vi "create.vi"(8 "error in (no error)":errorcluster, 10 "Port":i32, 11 "IModbusFactory in":refnum<class "IModbusFactory.lvclass">) -> (0 "error out":errorcluster, 2 "IModbus":refnum<class "IModbus.lvclass">, 3 "IModbusFactory out":refnum<class "IModbusFactory.lvclass">)   [LabVIEW 2016, in "IModbusFactory.lvclass"]
uses:
  IModbusFactory.lvclass
  IModbus/IModbus.lvclass
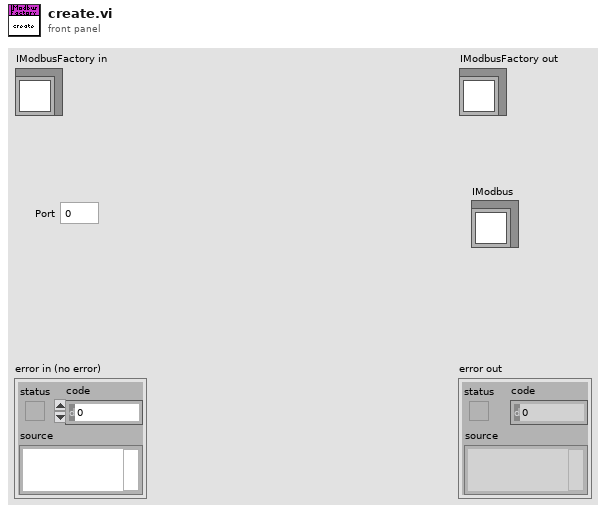
[diagram p1: front panel]
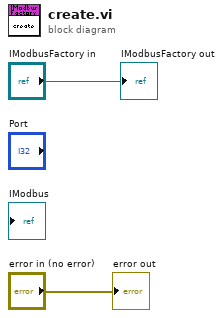
[diagram p0: block diagram]
diagram:
  "error out" <- "error in (no error)"
  "IModbusFactory out" <- "IModbusFactory in"
